vi "Test.vi"() -> ()   [LabVIEW 2018]
uses:
  PowerSupply4110/Type/SupplyConfig.ctl
  Controls/DataType.ctl
  PowerSupply4110/Type/SupplyOutput.ctl
panel:
  in  "Calibration":bool
  in  "Test Spec":T1={"PSU "={"Lower"=0.0002, "Upper"=1.0}, "Sensitivity"={"Lower"=0.2121, "Upper"=0.4243}, "THD"={"Lower"=1.0, "Upper"=0.0}}
  out "THD Mic2":dbl
  out "THD Mic1":dbl
  out "Sensitivity (mV/Pa) Mic2":dbl
  out "Processed Freq Response Mic1 2":cluster{dbl[], dbl[]}[](graph) caption="Fundamental-Response Mic1"
  out "Sensitivity (mV/Pa) Mic1":dbl
  out "Processed Freq Response Mic1":cluster{dbl[], dbl[]}[](graph) caption="Fundamental-Response Mic1"
  out "PLC\nCONNEC.":bool
  out "AUTO START\nCONDITION":bool
  out "Fundamental-Response 2":T2(graph) caption="Fundamental-Response Mic2"
  out "Fundamental-Response":T2(graph) caption="Fundamental-Response Mic1"
  in  "Adv 3":bool
  out "BUSY":bool
  out "AUTO RUN\nCOND.":bool
  out "JIG 1 CF":bool
  out "JIG 1 WS":bool
  in  "Label Print?":bool
  in  "Adv 2":bool
  in  "Adv":bool
  out "RESET":bool
  out "STOP":bool
  out "START":bool
  in  "Tab Control":enum32{"Response Level Mic1", "Page 2"}(tab)
  out "Current (mA)":dbl
  out "Voltage (V)":dbl
  out "THD-Response 2":cluster{"frequency":dbl[], "THD":dbl[]}(graph) caption="THD-Response"
  in  "OK Button":bool
  out "THD-Response":cluster{"frequency":dbl[], "THD":dbl[]}(graph)
  out "CHANNEL":bool
  out "ERROR":bool
  out "FAIL":bool
  out "PASS":bool
  out "FINISH":bool
  out "READY":bool
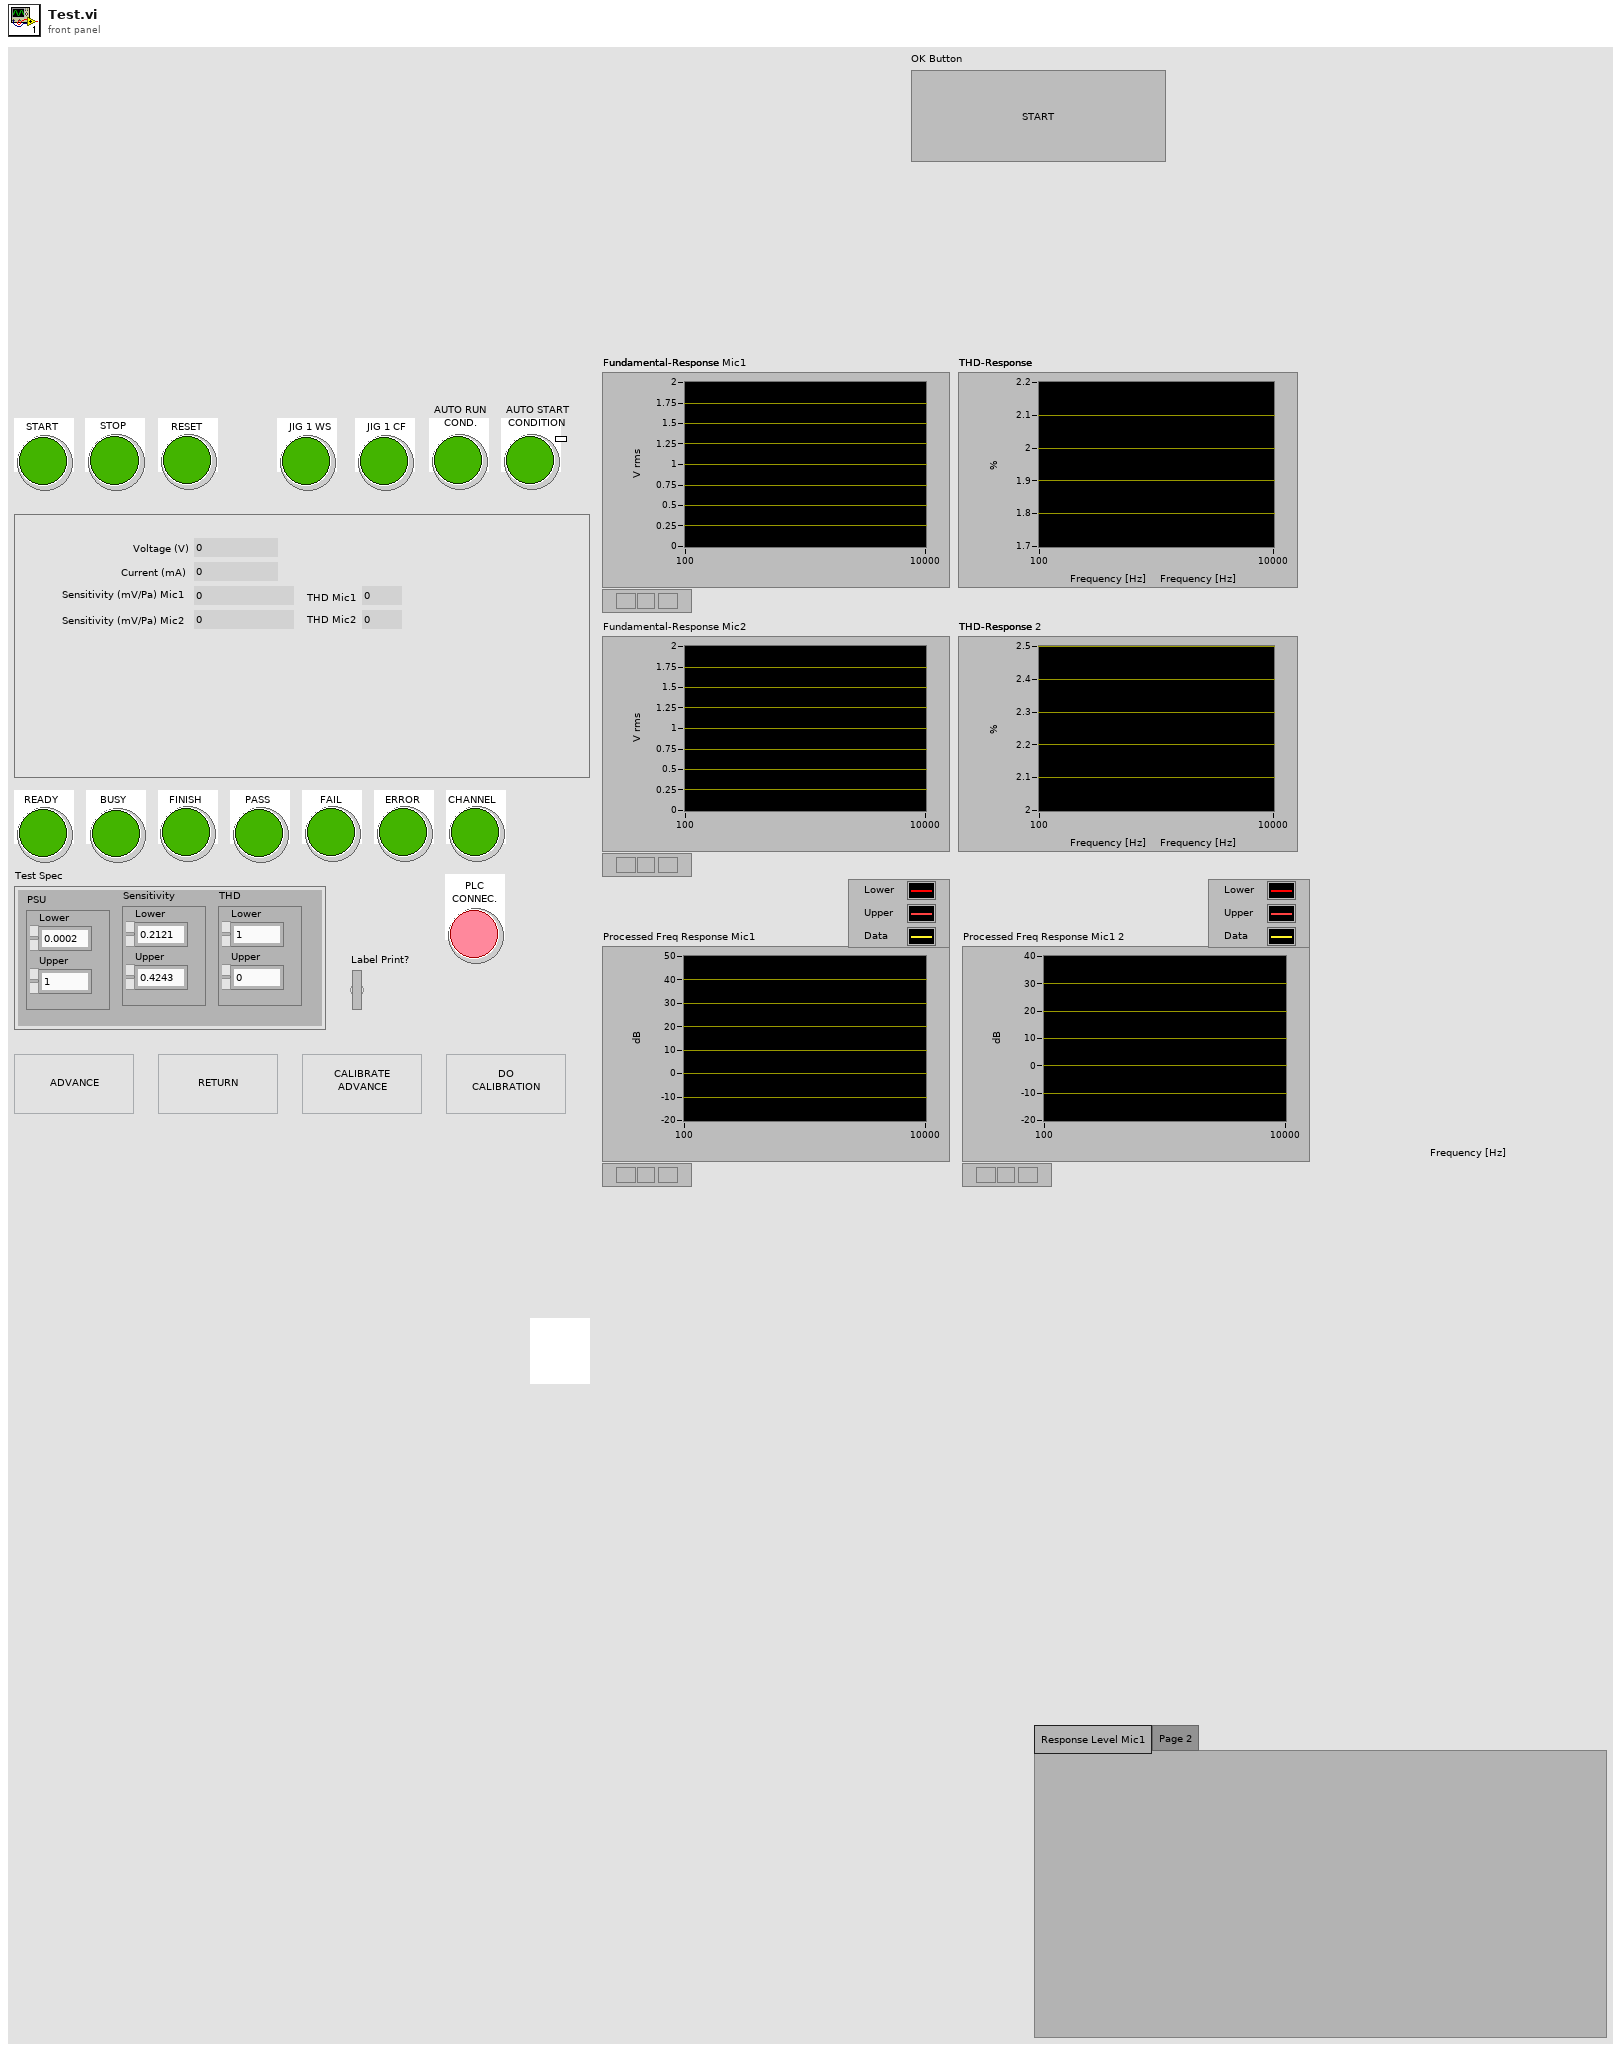
[diagram p1: front panel]
types:
  T1 = cluster{"PSU ":cluster{"Lower":dbl, "Upper":dbl}, "Sensitivity":cluster{"Lower":dbl, "Upper":dbl}, "THD":cluster{"Lower":dbl, "Upper":dbl}}
  T2 = cluster{"frequency [Hz]":dbl[], "amplitude":dbl[]}
  T3 = typedef "SupplyConfig.ctl" = cluster{"Channel Name":string, "Source Delay (Sec)":dbl, "Measurement:Sense":i32, "voltage level":dbl, "voltage level range":dbl, "current limit":dbl, "current limit range":dbl, "resource name":refnum<k15>}
  T4 = enum16{"Read", "Write", "ReadWrite", "BufferedRead", "BufferedReadWrite"}
  T5 = cluster{"frequency [Hz]":dbl, "amplitude [V]":dbl}[]
  T6 = typedef "DataType.ctl" = cluster{"Current":dbl, "Voltage":dbl, "Sensitivity":dbl, "THD":dbl, "FR":dbl[], "Sensitivity 2":dbl, "THD 2":dbl, "FR 2":dbl[]}
  T7 = typedef "SupplyOutput.ctl" = cluster{"Current max":dbl, "Current min":dbl, "Voltage max":dbl, "Voltage min":dbl, "Voltage mean":dbl, "Current mean":dbl}
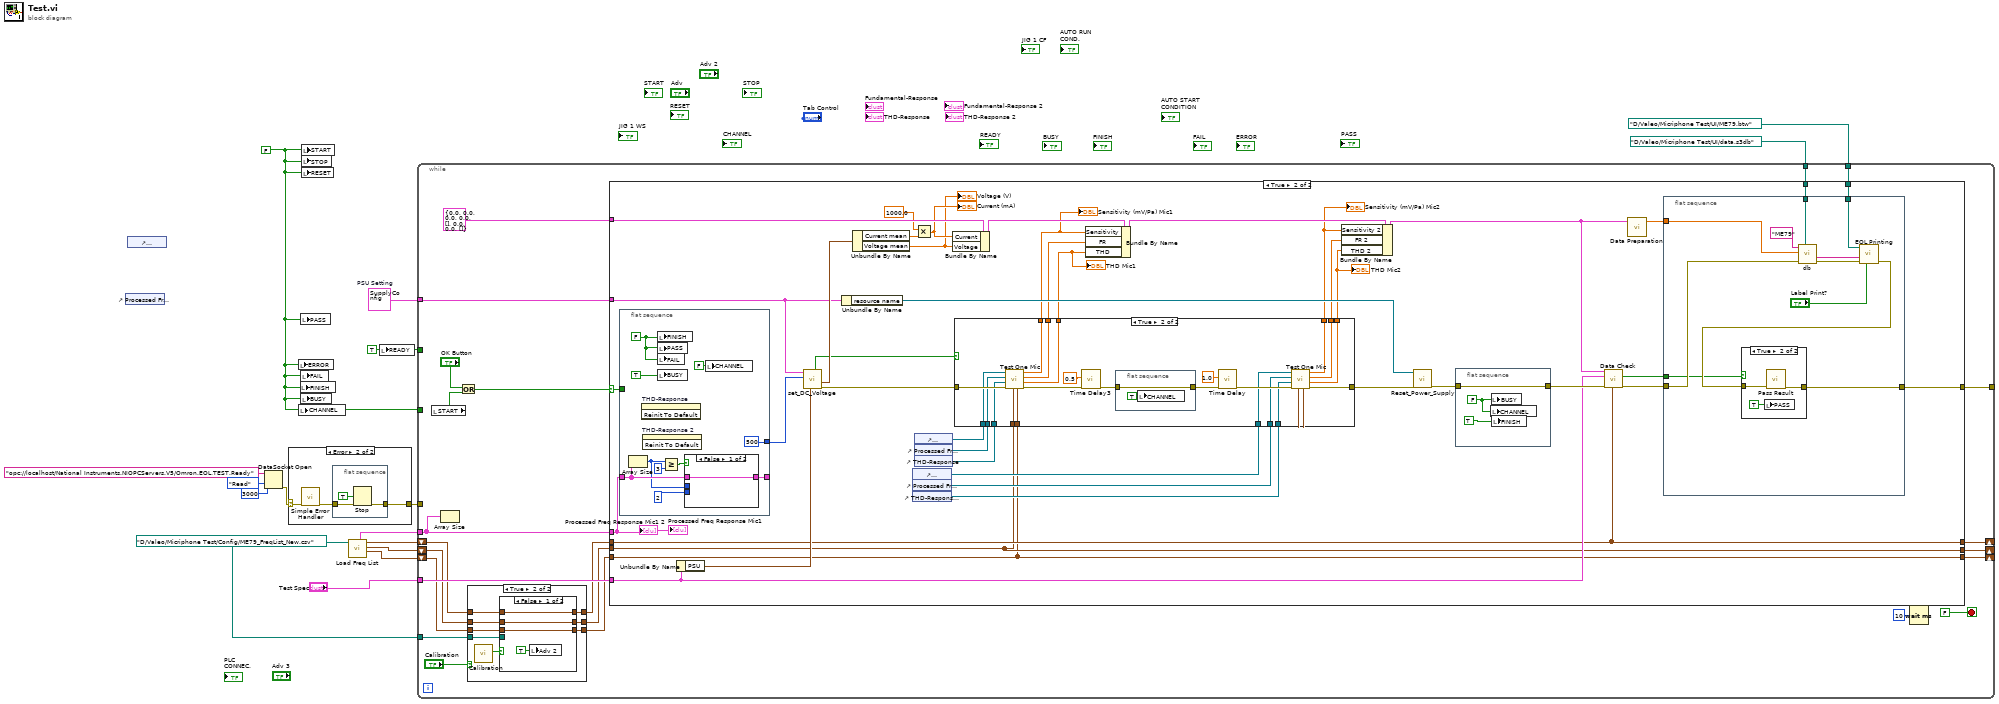
[diagram p0: block diagram]
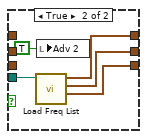
[diagram p4: hidden frame]
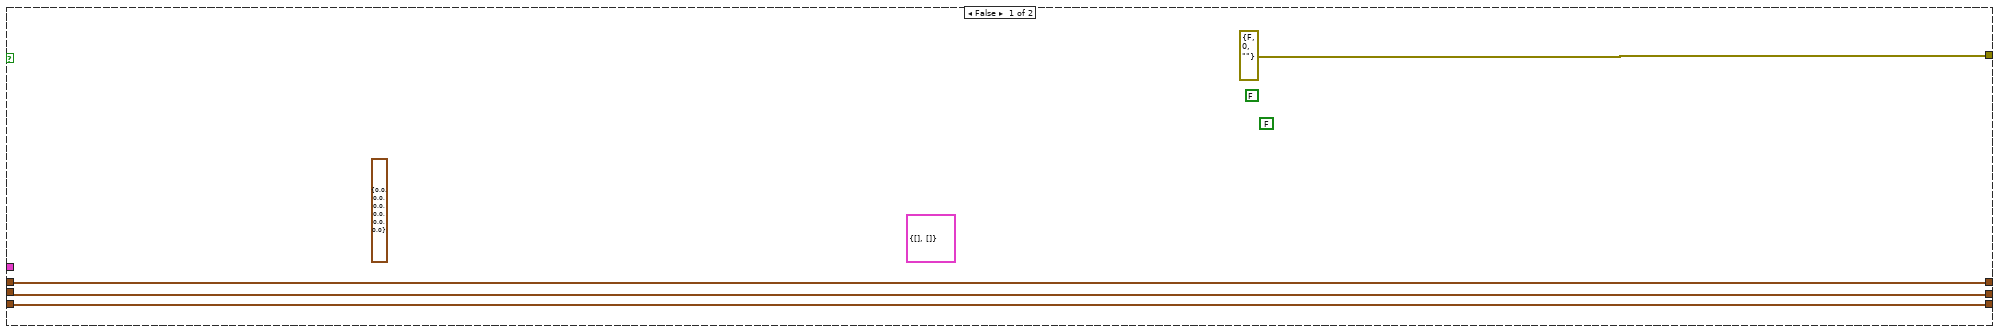
[diagram p5: hidden frame]
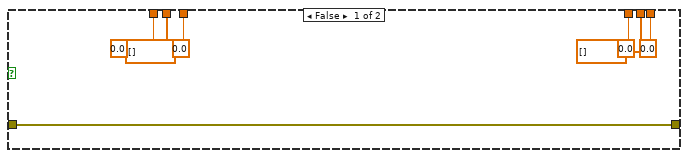
[diagram p6: hidden frame]
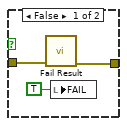
[diagram p7: hidden frame]
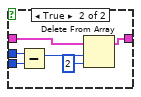
[diagram p8: hidden frame]
diagram:
  w9 = T3 {"Channel Name"="0", "Source Delay (Sec)"=1.0, "Measurement:Sense"=1008, "voltage level"=5.0, "voltage level range"=6.0, "current limit"=0.02, "current limit range"=0.02, "resource name"="PSU"}  # PSU Setting
  w4 = path "D:/Valeo/Micriphone Test/Config/ME79_FreqList_New.csv" ("Freq List file")
  w15 = FALSE
  w16 = TRUE ("Ready")
  n1 = control-ref of="Processed Freq Response Mic1"() -> ()  [unwired: 1 out]
  n2 = control-ref of="Fundamental-Response"() -> ()  [unwired: 1 out]
  n3 = DataSocket Open(9:3000 ("ms timeout (10000)"), 10:T4."Read" ("mode"), 11:"opc://localhost/National Instruments.NIOPCServers.V5/Omron.EOL.TEST.Ready" ("URL")) -> (0:w11:errorcluster)  [unwired: 1 in, 1 out]
  n4 = case shown="Error" w11 {
    selector: w11 -> [w17 w20]
    tunnel: [w17 w18] -> w10
    frame No Error {
    }
    frame Error {
      n5 = call <vilib>:"Simple Error Handler.vi"("error in (no error)"=w20) -> ("error out"=w19:errorcluster)  [unwired: 4 in, 4 out]
      n6 = flat-sequence {
        tunnel: w19 -> [w21]
        tunnel: [w21] -> w18
        frame #0 {
          n7 = Stop(stop? (T)=TRUE) -> ()
        }
      }
    }
  }
  n8 = local write "ERROR"(w15) -> ()
  n9 = local write "CHANNEL"(w15) -> ()
  n10 = local write "FINISH"(w15) -> ()
  n11 = local write "PASS"(w15) -> ()
  n12 = local write "FAIL"(w15) -> ()
  n13 = local write "BUSY"(w15) -> ()
  n14 = local write "START"(w15) -> ()
  n15 = local write "STOP"(w15) -> ()
  n16 = local write "RESET"(w15) -> ()
  n17 = call "Load Freq List.vi"("Freq List file"=w4) -> ("Freq for THD"=w1:cluster{"Numeric":dbl, "Numeric":dbl}[], "Frequency List"=w2:T5, "Spec List"=w3:cluster{"Lower":dbl, "Upper":dbl}[], "appended array"=w6:cluster{dbl[], dbl[]}[])  [unwired: 6 in, 1 out]
  n18 = local write "READY"(w16) -> ()
  n19 = while {
    tunnel: [w43] -> _
    tunnel: w16 -> [_]
    tunnel: w15 -> [_]
    tunnel: w10 -> [_]
    tunnel: w9 -> [w39]
    tunnel: path "D:/Valeo/Micriphone Test/UI/data.s3db" ("DB File") -> [w37]
    tunnel: path "D:/Valeo/Micriphone Test/UI/ME79.btw" ("Path") -> [w36]
    tunnel: w6 -> [w35]
    tunnel: "Test Spec" -> [w34]
    tunnel: w4 -> [w32]
    shift-right: [w25] -> _
    shift-left: w3 -> [w26]
    shift-right: [w24] -> _
    shift-left: w2 -> [w27]
    shift-right: [w23] -> _
    shift-left: w1 -> [w28]
    stop <- FALSE stop-if-true
    n20 = local read "START"() -> (w40:bool)
    n21 = Array Size(array=w35) -> ()  [unwired: 1 out]
    n22 = Or(x="OK Button", y=w40) -> (x .or. y?=w41:bool)
    n23 = case shown="True" "Calibration" {
      tunnel: w32 -> [_ w56]
      tunnel: w26 -> [w48 w54]
      tunnel: w27 -> [w47 w53]
      tunnel: w28 -> [w46 w52]
      tunnel: [w48 w51] -> w29
      tunnel: [w47 w50] -> w30
      tunnel: [w46 w49] -> w31
      frame False {
      }
      frame True {
        n24 = call "Calibration.vi"() -> ("Cal Success"=w55:bool)  [unwired: 10 in, 1 out]
        n25 = case shown="False" w55 {
          tunnel: w56 -> [_ w65]
          tunnel: [w60 w64] -> w51
          tunnel: w54 -> [w60 _]
          tunnel: [w59 w63] -> w50
          tunnel: w53 -> [w59 _]
          tunnel: [w58 w62] -> w49
          tunnel: w52 -> [w58 _]
          frame False {
            n26 = local write "Adv 2"(TRUE ("Adv 2")) -> ()
          }
          frame True {
            n27 = call "Load Freq List.vi"("Freq List file"=w65) -> ("Freq for THD"=w62:cluster{"Numeric":dbl, "Numeric":dbl}[], "Frequency List"=w63:T5, "Spec List"=w64:cluster{"Lower":dbl, "Upper":dbl}[])  [unwired: 6 in, 2 out]
            n28 = local write "Adv 2"(TRUE ("Adv 2")) -> ()
          }
        }
      }
    }
    n29 = case shown="True" w41 {
      selector: w41 -> [_ w104]
      tunnel: [errorcluster {"status"=FALSE, "code"=0, "source"=""} ("error out") w109] -> w43
      tunnel: T6 {"Current"=0.0, "Voltage"=0.0, "Sensitivity"=0.0, "THD"=0.0, "FR"=[], "Sensitivity 2"=0.0, "THD 2"=0.0, "FR 2"=[]} ("Data") -> [_ w107]
      tunnel: w30 -> [w67 w71]
      tunnel: w31 -> [w66 w70]
      tunnel: w39 -> [_ w103]
      tunnel: w37 -> [_ w101]
      tunnel: w36 -> [_ w100]
      tunnel: w29 -> [w68 w72]
      tunnel: w35 -> [_ w97]
      tunnel: w34 -> [_ w76]
      tunnel: [w68 w72] -> w25
      tunnel: [w67 w71] -> w24
      tunnel: [w66 w70] -> w23
      frame False {
        (unwired) T7 {"Current max"=0.0, "Current min"=0.0, "Voltage max"=0.0, "Voltage min"=0.0, "Voltage mean"=0.0, "Current mean"=0.0} ("Supply Output")
        (unwired) cluster{"frequency":dbl[], "magnitude":dbl[]} {"frequency"=[], "magnitude"=[]} ("Response Level")
        (unwired) FALSE ("Busy")
        (unwired) FALSE ("Busy")
      }
      frame True {
        n30 = flat-sequence {
          tunnel: [500 ("Messdauer/ms")] -> w108
          tunnel: w104 -> [_]
          tunnel: w97 -> [w164]
          tunnel: [w161] -> _
          frame #0 {
            w168 = FALSE ("Finish")
            n31 = Array Size(array=w164) -> (size(s)=w163:i32)
            n32 = invoke on="THD-Response" class="XYGraph (strict)" method="Reinit To Default"() -> ()  [unwired: 3 in, 3 out]
            n33 = invoke on="THD-Response 2" class="XYGraph (strict)" method="Reinit To Default"() -> ()  [unwired: 3 in, 3 out]
            n34 = local write "FINISH"(w168) -> ()
            n35 = local write "PASS"(w168) -> ()
            n36 = local write "FAIL"(w168) -> ()
            n37 = local write "BUSY"(TRUE ("Finish")) -> ()
            n38 = Greater Or Equal?(x=w163, y=3) -> (x >= y?=w165:bool)
            n39 = case shown="False" w165 {
              tunnel: w164 -> [w170 w176]
              tunnel: w163 -> [_ w175]
              tunnel: 2 ("y") -> [_ w174]
              tunnel: [w170 w171] -> w161
              frame False {
              }
              frame True {
                n40 = Subtract(x=w175, y=w174) -> (x-y=w173:i32)
                n41 = Delete From Array(array=w176, length=w173, index=2) -> (array with subset deleted=w171:cluster{dbl[], dbl[]}[])  [unwired: 1 out]
              }
            }
            n42 = local write "CHANNEL"(FALSE ("Channel")) -> ()
          }
        }
        n43 = Unbundle By Name(w76) -> ("PSU"=w77:cluster{"Lower":dbl, "Upper":dbl})
        n44 = call "set_DC_Voltage.vi"("PSU Spec"=w77, "Messdauer/ms"=w108, "Einstellungen"=w103) -> ("error out"=w96:errorcluster, "Supply Output"=w106:T7, "PSU OK?"=w81:bool)  [unwired: 4 in, 2 out]
        n45 = Unbundle By Name(w103) -> ("resource name"=w111:refnum<k15>)
        n46 = Unbundle By Name(w106) -> ("Current mean"=w99:dbl, "Voltage mean"=w73:dbl)
        "Voltage (V)" <- w73
        n47 = control-ref of="Fundamental-Response 2"() -> (w88:refnum<vi>)
        n48 = control-ref of="Processed Freq Response Mic1 2"() -> (w87:refnum<vi>)
        n49 = control-ref of="THD-Response 2"() -> (w86:refnum<vi>)
        n50 = control-ref of="Fundamental-Response"() -> (w95:refnum<vi>)
        n51 = control-ref of="Processed Freq Response Mic1"() -> (w94:refnum<vi>)
        n52 = control-ref of="THD-Response"() -> (w93:refnum<vi>)
        n53 = Multiply(x=1000.0 ("y"), y=w99) -> (x*y=w74:dbl)
        "Current (mA)" <- w74
        n54 = Bundle By Name(cluster=w107, "Current"=w74, "Voltage"=w73) -> (w105:T6)
        n55 = case shown="True" w81 {
          tunnel: w96 -> [w112 w137]
          tunnel: w95 -> [_ w136]
          tunnel: w94 -> [_ w135]
          tunnel: w93 -> [_ w134]
          tunnel: [0.0 ("Sensitivity (dBSPL)") w132] -> w92
          tunnel: [dbl[] [] ("ProcessedFrequencyResponse") w131] -> w91
          tunnel: [0.0 ("THD") w129] -> w89
          tunnel: w88 -> [_ w127]
          tunnel: w87 -> [_ w126]
          tunnel: w86 -> [_ w125]
          tunnel: [dbl[] [] ("ProcessedFrequencyResponse") w124] -> w85
          tunnel: w71 -> [_ w123]
          tunnel: w70 -> [_ w122]
          tunnel: [0.0 ("Sensitivity (dBSPL)") w121] -> w84
          tunnel: [w112 w120] -> w83
          tunnel: [0.0 ("THD") w119] -> w82
          frame False {
          }
          frame True {
            n56 = call "Test One Mic.vi"("Freq for THD"=w122, "Frequency List"=w123, "error in (no error)"=w137, "THD-Response"=w134, "Freq Response Mic1"=w135, "Response1"=w136) -> ("error out"=w133:errorcluster, "THD"=w129:dbl, "ProcessedFrequencyResponse"=w131:dbl[], "Sensitivity (dBSPL)"=w132:dbl)  [unwired: 2 in]
            n57 = call "Time Delay3"("error in (no error)"=w133, "Delay Time (s)"=0.5) -> ("error out"=w130:errorcluster)  [unwired: 9 in]
            n58 = flat-sequence {
              tunnel: w130 -> [w142]
              tunnel: [w142] -> w140
              frame #0 {
                n59 = local write "CHANNEL"(TRUE ("Channel")) -> ()
              }
            }
            n60 = call "Time Delay"("error in (no error)"=w140, "Delay Time (s)"=1.0) -> ("error out"=w128:errorcluster)  [unwired: 9 in]
            n61 = call "Test One Mic.vi"("Freq for THD"=w122, "Frequency List"=w123, "error in (no error)"=w128, "THD-Response"=w125, "Freq Response Mic1"=w126, "Response1"=w127) -> ("error out"=w120:errorcluster, "THD"=w119:dbl, "ProcessedFrequencyResponse"=w124:dbl[], "Sensitivity (dBSPL)"=w121:dbl)  [unwired: 2 in]
          }
        }
        "Sensitivity (mV/Pa) Mic2" <- w84
        "Sensitivity (mV/Pa) Mic1" <- w92
        "THD Mic1" <- w89
        "THD Mic2" <- w82
        n62 = Bundle By Name(cluster=w105, "Sensitivity"=w92, "FR"=w91, "THD"=w89) -> (w90:T6)
        n63 = Bundle By Name(cluster=w90, "Sensitivity 2"=w84, "FR 2"=w85, "THD 2"=w82) -> (w78:T6)
        n64 = call "Reset_Power_Supply.vi"("error in (no error)"=w83, "resource name"=w111) -> ("error out"=w110:errorcluster)  [unwired: 9 in]
        n65 = flat-sequence {
          tunnel: w110 -> [w179]
          tunnel: [w179] -> w80
          frame #0 {
            w177 = FALSE ("Channel")
            n66 = local write "CHANNEL"(w177) -> ()
            n67 = local write "BUSY"(w177) -> ()
            n68 = local write "FINISH"(TRUE ("Busy")) -> ()
          }
        }
        n69 = call "Data Check.vi"("Spec List"=w72, "error in (no error)"=w80, "Test Spec"=w76, "Data"=w78) -> ("error out"=w79:errorcluster, "All Result"=w75:bool)  [unwired: 6 in]
        n70 = call "Data Preparation.vi"("Data"=w78) -> ("Measured Data Out"=w102:dbl[])  [unwired: 4 in]
        n71 = flat-sequence {
          tunnel: w79 -> [w151]
          tunnel: [w143] -> w109
          tunnel: w102 -> [w152]
          tunnel: w101 -> [w150]
          tunnel: w100 -> [w147]
          tunnel: w75 -> [w144]
          frame #0 {
            n72 = call "db.vi"("DB File"=w150, "error in (no error)"=w151, "Datas In"=w152, "Model"="ME79") -> ("error out"=w149:errorcluster, "SN Out"=w148:string)  [unwired: 5 in, 1 out]
            n73 = call "EOL Printing.vi"("Print?"="Label Print?", "error in (no error)"=w149, "DATA"=w148, "Path"=w147) -> ("error out"=w145:errorcluster)  [unwired: 7 in]
            n74 = case shown="True" w144 {
              tunnel: w145 -> [w156 w159]
              tunnel: [w155 w158] -> w143
              frame False {
                n75 = call "Fail Result.vi"("error in (no error)"=w156) -> ("error out"=w155:errorcluster)  [unwired: 10 in]
                n76 = local write "FAIL"(TRUE ("FAIL")) -> ()
              }
              frame True {
                n77 = local write "PASS"(TRUE ("PASS")) -> ()
                n78 = call "Pass Result.vi"("error in (no error)"=w159) -> ("error out"=w158:errorcluster)  [unwired: 10 in]
              }
            }
          }
        }
        "Processed Freq Response Mic1 2" <- w97
        "Processed Freq Response Mic1" <- w97
      }
    }
    n79 = Wait (ms)(milliseconds to wait=u32 10) -> ()  [unwired: 1 out]
  }
